vi "MotorLaserScan.vi"() -> ()   [LabVIEW 2017]
panel:
  in  "Step size Y (mm)":dbl=0.2
  in  "Initial Y (mm)":dbl=7.1
  in  "Final Y (mm)":dbl=11.3
  in  "Y Motor Control":refnum<k7>(container)
  in  "Step size (mm)":dbl=0.02
  in  "X Motor Control":refnum<k7>(container)
  in  "Final (mm)":dbl=20.0
  in  "Initial (mm)":dbl=13.4
  # "Laser Scan Motor Control Program"
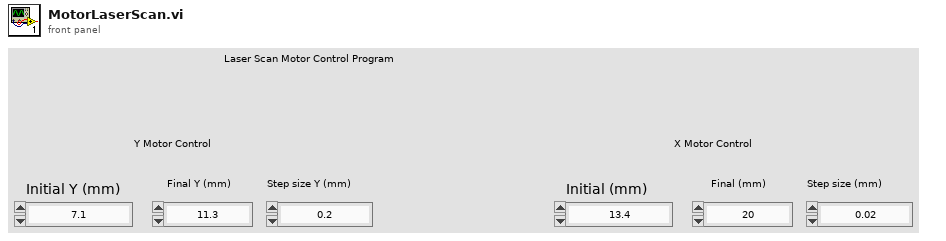
[diagram p1: front panel]
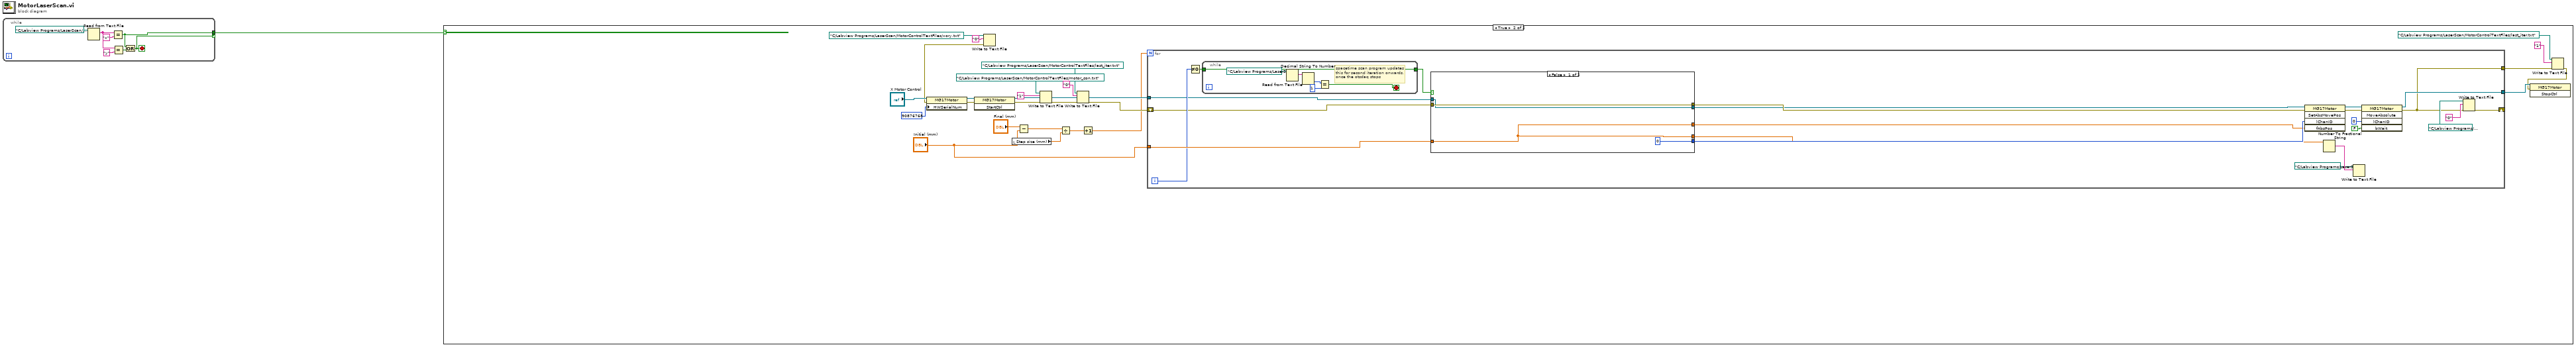
[diagram p0: block diagram]
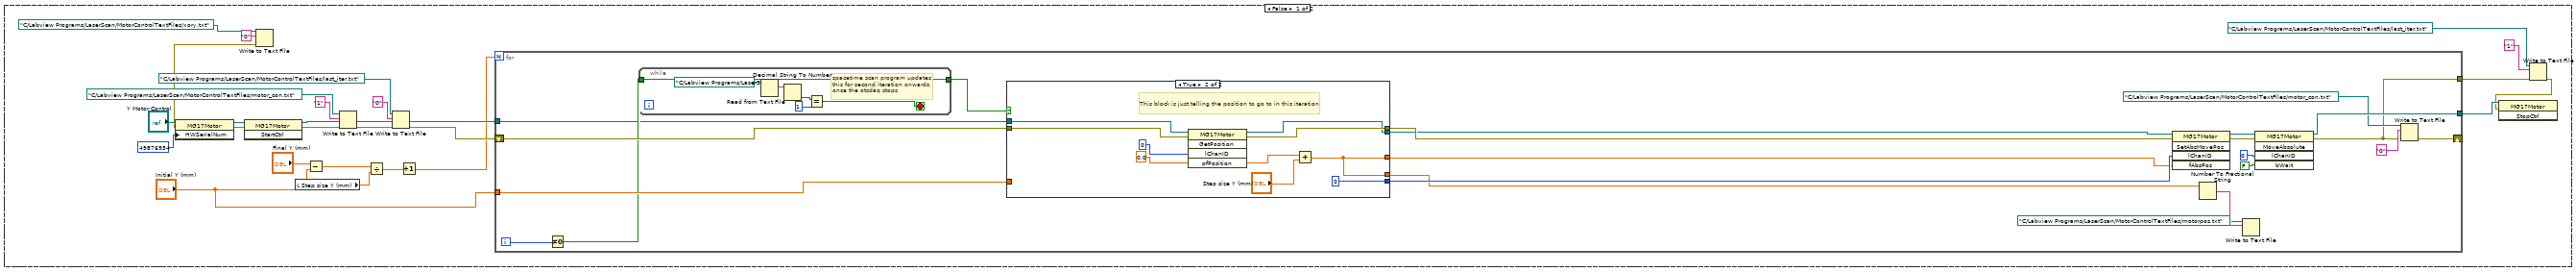
[diagram p2: hidden frame]
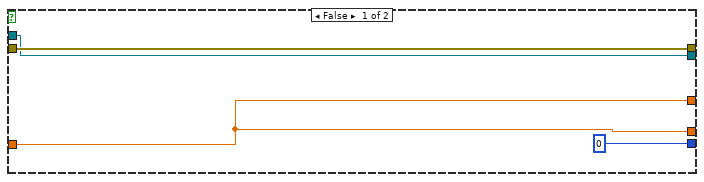
[diagram p3: hidden frame]
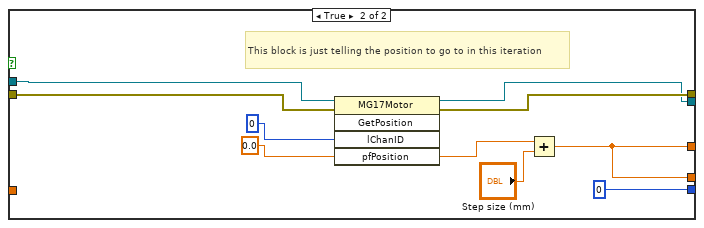
[diagram p4: hidden frame]
diagram:
  n1 = while {
    tunnel: [w4] -> w1 if=w2
    stop <- w2 stop-if-true
    n2 = Read from Text File(file (use dialog)=path "C:/Labview Programs/LaserScan/MotorControlTextFiles/xory.txt") -> (text=w5:string)  [unwired: 3 in, 3 out]
    n3 = Equal?(x=w5, y="x") -> (x = y?=w4:bool)
    n4 = Equal?(x=w5, y="y") -> (x = y?=w3:bool)
    n5 = Or(x=w4, y=w3) -> (x .or. y?=w2:bool)
  }
  n6 = case shown="True" w1 {
    frame False {
      n7 = Write to Text File(file (use dialog)=path "C:/Labview Programs/LaserScan/MotorControlTextFiles/xory.txt" ("file path (use dialog)"), text="0") -> (error out=w15:errorcluster)  [unwired: 2 in, 2 out]
      n8 = property class="MG17Motor"(reference="Y Motor Control", error in=w15, "HWSerialNum"=49876934 ("Serial")) -> (reference out=w32:refnum<k7>, error out=w30:errorcluster)
      n9 = invoke class="MG17Motor" method="StartCtrl"(reference=w32, error in=w30) -> (reference out=w29:refnum<k7>, error out=w23:errorcluster)  [unwired: 1 in, 1 out]
      n10 = local read "Step size Y (mm)"() -> (w22:dbl)
      n11 = Subtract(x="Final Y (mm)", y="Initial Y (mm)") -> (x-y=w28:dbl)
      n12 = Write to Text File(file (use dialog)=path "C:/Labview Programs/LaserScan/MotorControlTextFiles/motor_con.txt" ("file path (use dialog)"), text="1", error in=w23) -> (error out=w19:errorcluster)  [unwired: 1 in, 2 out]
      n13 = Divide(x=w28, y=w22) -> (x/y=w10:dbl)
      n14 = Write to Text File(file (use dialog)=path "C:/Labview Programs/LaserScan/MotorControlTextFiles/last_iter.txt" ("file path (use dialog)"), text="0", error in=w19) -> (error out=w18:errorcluster)  [unwired: 1 in, 2 out]
      n15 = Increment(x=w10) -> (x+1=w9:dbl)
      n16 = for {
        N: w9 -> [_]
        tunnel: [w50] -> w31
        tunnel: w29 -> [w37]
        tunnel: "Initial Y (mm)" -> [w47]
        shift-right: [w40] -> _
        shift-left: w18 -> [w41]
        tunnel: [w35] -> w14
        i -> [w42]
        n17 = Not Equal To 0?(x=w42) -> (x != 0?=w39:bool)
        n18 = while {
          tunnel: w39 -> [w57]
          tunnel: [w57] -> w38
          stop <- w58 stop-if-true
          # "spacetime scan program updates this for second iteration onwards, once the otsdaq stops"
          n19 = Read from Text File(file (use dialog)=path "C:/Labview Programs/LaserScan/MotorControlTextFiles/motor_con.txt") -> (text=w61:string)  [unwired: 3 in, 3 out]
          n20 = Decimal String To Number(string=w61) -> (number=w60:i32)  [unwired: 2 in, 1 out]
          n21 = Equal?(x=w60, y=1) -> (x = y?=w58:bool)
        }
        n22 = case shown="True" w38 {
          tunnel: [0 ("lChanID") 0 ("lChanID")] -> w56
          tunnel: [w64 w69] -> w52
          tunnel: w41 -> [w66 w75]
          tunnel: [w66 w72] -> w49
          tunnel: w47 -> [w64 _]
          tunnel: [w64 w69] -> w46
          tunnel: w37 -> [w63 w68]
          tunnel: [w63 w67] -> w36
          frame False {
          }
          frame True {
            # "This block is just telling the position to go to in this iteration"
            n23 = invoke class="MG17Motor" method="GetPosition"(reference=w68, error in=w75, "lChanID"=0, "pfPosition"=sgl 0.0) -> (reference out=w67:refnum<k7>, error out=w72:errorcluster, "pfPosition"=w71:sgl)  [unwired: 1 in, 2 out]
            n24 = Add(x=w71, y="Step size Y (mm)") -> (x+y=w69:dbl)
          }
        }
        n25 = invoke class="MG17Motor" method="SetAbsMovePos"(reference=w36, error in=w49, "lChanID"=w56, "fAbsPos"=w52) -> (reference out=w54:refnum<k7>, error out=w51:errorcluster)  [unwired: 1 in, 3 out]
        n26 = Number To Fractional String(number=w46) -> (F-format string=w45:string)  [unwired: 3 in]
        n27 = Write to Text File(file (use dialog)=path "C:/Labview Programs/LaserScan/MotorControlTextFiles/motorpos.txt" ("file path (use dialog)"), text=w45) -> ()  [unwired: 2 in, 3 out]
        n28 = invoke class="MG17Motor" method="MoveAbsolute"(reference=w54, error in=w51, "lChanID"=0, "bWait"=FALSE ("bWait 2")) -> (reference out=w50:refnum<k7>, error out=w35:errorcluster)  [unwired: 1 in, 3 out]
        n29 = Write to Text File(file (use dialog)=path "C:/Labview Programs/LaserScan/MotorControlTextFiles/motor_con.txt" ("file path (use dialog)"), text="0", error in=w35) -> (error out=w40:errorcluster)  [unwired: 1 in, 2 out]
      }
      n30 = Write to Text File(file (use dialog)=path "C:/Labview Programs/LaserScan/MotorControlTextFiles/last_iter.txt" ("file path (use dialog)"), text="1", error in=w14) -> (error out=w12:errorcluster)  [unwired: 1 in, 2 out]
      n31 = invoke class="MG17Motor" method="StopCtrl"(reference=w31, error in=w12) -> ()  [unwired: 1 in, 3 out]
    }
    frame True {
      n32 = Write to Text File(file (use dialog)=path "C:/Labview Programs/LaserScan/MotorControlTextFiles/xory.txt" ("file path (use dialog)"), text="0") -> (error out=w83:errorcluster)  [unwired: 2 in, 2 out]
      n33 = property class="MG17Motor"(reference="X Motor Control", error in=w83, "HWSerialNum"=90876768 ("Serial")) -> (reference out=w100:refnum<k7>, error out=w98:errorcluster)
      n34 = invoke class="MG17Motor" method="StartCtrl"(reference=w100, error in=w98) -> (reference out=w97:refnum<k7>, error out=w91:errorcluster)  [unwired: 1 in, 1 out]
      n35 = local read "Step size (mm)"() -> (w90:dbl)
      n36 = Subtract(x="Final (mm)", y="Initial (mm)") -> (x-y=w96:dbl)
      n37 = Write to Text File(file (use dialog)=path "C:/Labview Programs/LaserScan/MotorControlTextFiles/motor_con.txt" ("file path (use dialog)"), text="1", error in=w91) -> (error out=w87:errorcluster)  [unwired: 1 in, 2 out]
      n38 = Divide(x=w96, y=w90) -> (x/y=w78:dbl)
      n39 = Write to Text File(file (use dialog)=path "C:/Labview Programs/LaserScan/MotorControlTextFiles/last_iter.txt" ("file path (use dialog)"), text="0", error in=w87) -> (error out=w86:errorcluster)  [unwired: 1 in, 2 out]
      n40 = Increment(x=w78) -> (x+1=w77:dbl)
      n41 = for {
        N: w77 -> [_]
        tunnel: [w118] -> w99
        tunnel: w97 -> [w105]
        tunnel: "Initial (mm)" -> [w115]
        shift-right: [w108] -> _
        shift-left: w86 -> [w109]
        tunnel: [w103] -> w82
        i -> [w110]
        n42 = Not Equal To 0?(x=w110) -> (x != 0?=w107:bool)
        n43 = while {
          tunnel: w107 -> [w125]
          tunnel: [w125] -> w106
          stop <- w126 stop-if-true
          # "spacetime scan program updates this for second iteration onwards, once the otsdaq stops"
          n44 = Read from Text File(file (use dialog)=path "C:/Labview Programs/LaserScan/MotorControlTextFiles/motor_con.txt") -> (text=w129:string)  [unwired: 3 in, 3 out]
          n45 = Decimal String To Number(string=w129) -> (number=w128:i32)  [unwired: 2 in, 1 out]
          n46 = Equal?(x=w128, y=1) -> (x = y?=w126:bool)
        }
        n47 = case shown="False" w106 {
          tunnel: [0 ("lChanID") 0 ("lChanID")] -> w124
          tunnel: [w132 w137] -> w120
          tunnel: w109 -> [w134 w143]
          tunnel: [w134 w140] -> w117
          tunnel: w115 -> [w132 _]
          tunnel: [w132 w137] -> w114
          tunnel: w105 -> [w131 w136]
          tunnel: [w131 w135] -> w104
          frame False {
          }
          frame True {
            # "This block is just telling the position to go to in this iteration"
            n48 = invoke class="MG17Motor" method="GetPosition"(reference=w136, error in=w143, "lChanID"=0, "pfPosition"=sgl 0.0) -> (reference out=w135:refnum<k7>, error out=w140:errorcluster, "pfPosition"=w139:sgl)  [unwired: 1 in, 2 out]
            n49 = Add(x=w139, y="Step size (mm)") -> (x+y=w137:dbl)
          }
        }
        n50 = invoke class="MG17Motor" method="SetAbsMovePos"(reference=w104, error in=w117, "lChanID"=w124, "fAbsPos"=w120) -> (reference out=w122:refnum<k7>, error out=w119:errorcluster)  [unwired: 1 in, 3 out]
        n51 = Number To Fractional String(number=w114) -> (F-format string=w113:string)  [unwired: 3 in]
        n52 = Write to Text File(file (use dialog)=path "C:/Labview Programs/LaserScan/MotorControlTextFiles/motorpos.txt" ("file path (use dialog)"), text=w113) -> ()  [unwired: 2 in, 3 out]
        n53 = invoke class="MG17Motor" method="MoveAbsolute"(reference=w122, error in=w119, "lChanID"=0, "bWait"=FALSE ("bWait 2")) -> (reference out=w118:refnum<k7>, error out=w103:errorcluster)  [unwired: 1 in, 3 out]
        n54 = Write to Text File(file (use dialog)=path "C:/Labview Programs/LaserScan/MotorControlTextFiles/motor_con.txt" ("file path (use dialog)"), text="0", error in=w103) -> (error out=w108:errorcluster)  [unwired: 1 in, 2 out]
      }
      n55 = Write to Text File(file (use dialog)=path "C:/Labview Programs/LaserScan/MotorControlTextFiles/last_iter.txt" ("file path (use dialog)"), text="1", error in=w82) -> (error out=w80:errorcluster)  [unwired: 1 in, 2 out]
      n56 = invoke class="MG17Motor" method="StopCtrl"(reference=w99, error in=w80) -> ()  [unwired: 1 in, 3 out]
    }
  }
